vi "Write instrumentName.vi"(8 "error in (no error)":errorcluster, 10 "instrumentName":string, 11 "instrumentSelect in":refnum<class "InstrumentSelect.lvclass">) -> (0 "error out":errorcluster, 3 "instrumentSelect out":refnum<class "InstrumentSelect.lvclass">)   [LabVIEW 2022 SP3, in "TCSDataDefinitions.lvlib" / "TCSCommand.lvlib" / "InstrumentSelect.lvclass"]
uses:
  InstrumentSelect.lvclass
  InstrumentSelect.lvclass/InstrumentSelect.ctl
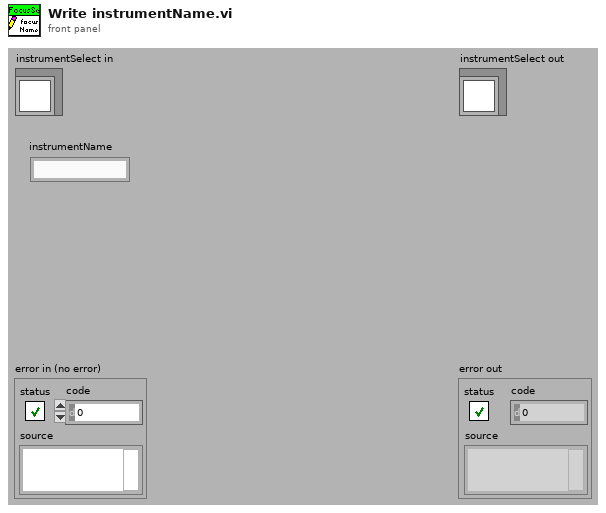
[diagram p1: front panel]
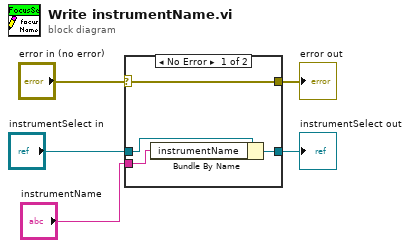
[diagram p0: block diagram]
diagram:
  n1 = case shown="No Error" "error in (no error)" {
    selector: "error in (no error)" -> [w9 w10]
    tunnel: [w9 w10] -> w4
    tunnel: [w7 w11] -> w2
    tunnel: "instrumentSelect in" -> [w8 w11]
    tunnel: "instrumentName" -> [w6 _]
    frame No Error {
      n2 = Bundle By Name(cluster=w8, "instrumentName"=w6) -> (w7:refnum<class "InstrumentSelect.lvclass">)
    }
    frame Error {
    }
  }
  "error out" <- w4
  "instrumentSelect out" <- w2
